vi "Event-Window.vi"(8 "error in (no error)":errorcluster, 9 "WindowEvent":T2, 10 "EventType":T1=enum."SDL_EVENT_WINDOW_DESTROYED", 11 "DVR Cluster In":T4={"CMD Queue"=refnum, "Config"={"Quit On Last Window Closed"=FALSE, "VSync"=enum."Disabled", "FPS Target"=30.0}, "Ctxt"={"VSync Enabled"=FALSE}, "Metrics"={"Uptime [ms]"=0, "Loop Time [ms]"=0, "Timer [ns]"=0, "Poll Events [ns]"=0, "Dequeue CMD [ns]"=0, "Update Layout [ns]"=0, "Render [ns]"=0}, "Debug"={"Unhandled Events"={}}, "ID To Window"={}, "Window To Handle"={}, "Event Interface"=refnum}) -> (0 "error out":errorcluster, 3 "DVR Cluster Out":T4={"CMD Queue"=refnum, "Config"={"Quit On Last Window Closed"=FALSE, "VSync"=enum."Disabled", "FPS Target"=30.0}, "Ctxt"={"VSync Enabled"=FALSE}, "Metrics"={"Uptime [ms]"=0, "Loop Time [ms]"=0, "Timer [ns]"=0, "Poll Events [ns]"=0, "Dequeue CMD [ns]"=0, "Update Layout [ns]"=0, "Render [ns]"=0}, "Debug"={"Unhandled Events"={}}, "ID To Window"={}, "Window To Handle"={}, "Event Interface"=refnum})   [LabVIEW 2020, in "GLF.lvlib" / "Engine.lvclass"]
uses:
  Engine.lvclass
  EngineEventInterface/EngineEventInterface.lvclass
  Window/Window.lvclass
  Engine.lvclass/Engine.ctl
  <vilib>/Utility/miscctls.llb/LVMapReplaceAction.ctl
  <vilib>/Saukko/LV SDL3/Sources/SDL3/Events/EventType--enum.ctl
  <vilib>/Saukko/LV SDL3/Sources/SDL3/Events/Events.lvlib
  <vilib>/Saukko/LV SDL3/Sources/SDL3/Video/DisplayID--integer.ctl
  <vilib>/Saukko/LV SDL3/Sources/SDL3/Video/Video.lvlib
  VSync--enum.ctl
  Config--cluster.ctl
  Context--cluster.ctl
  Metrics--cluster.ctl
  Command--enum.ctl
  Command--cluster.ctl
  Command--queue.ctl
  <vilib>/Saukko/LV SDL3/Sources/SDL3/Video/WindowID--integer.ctl
  DVR--cluster.ctl
  <vilib>/Saukko/LV SDL3/Sources/SDL3/Events/WindowEventData--cluster.ctl
  Debug--cluster.ctl
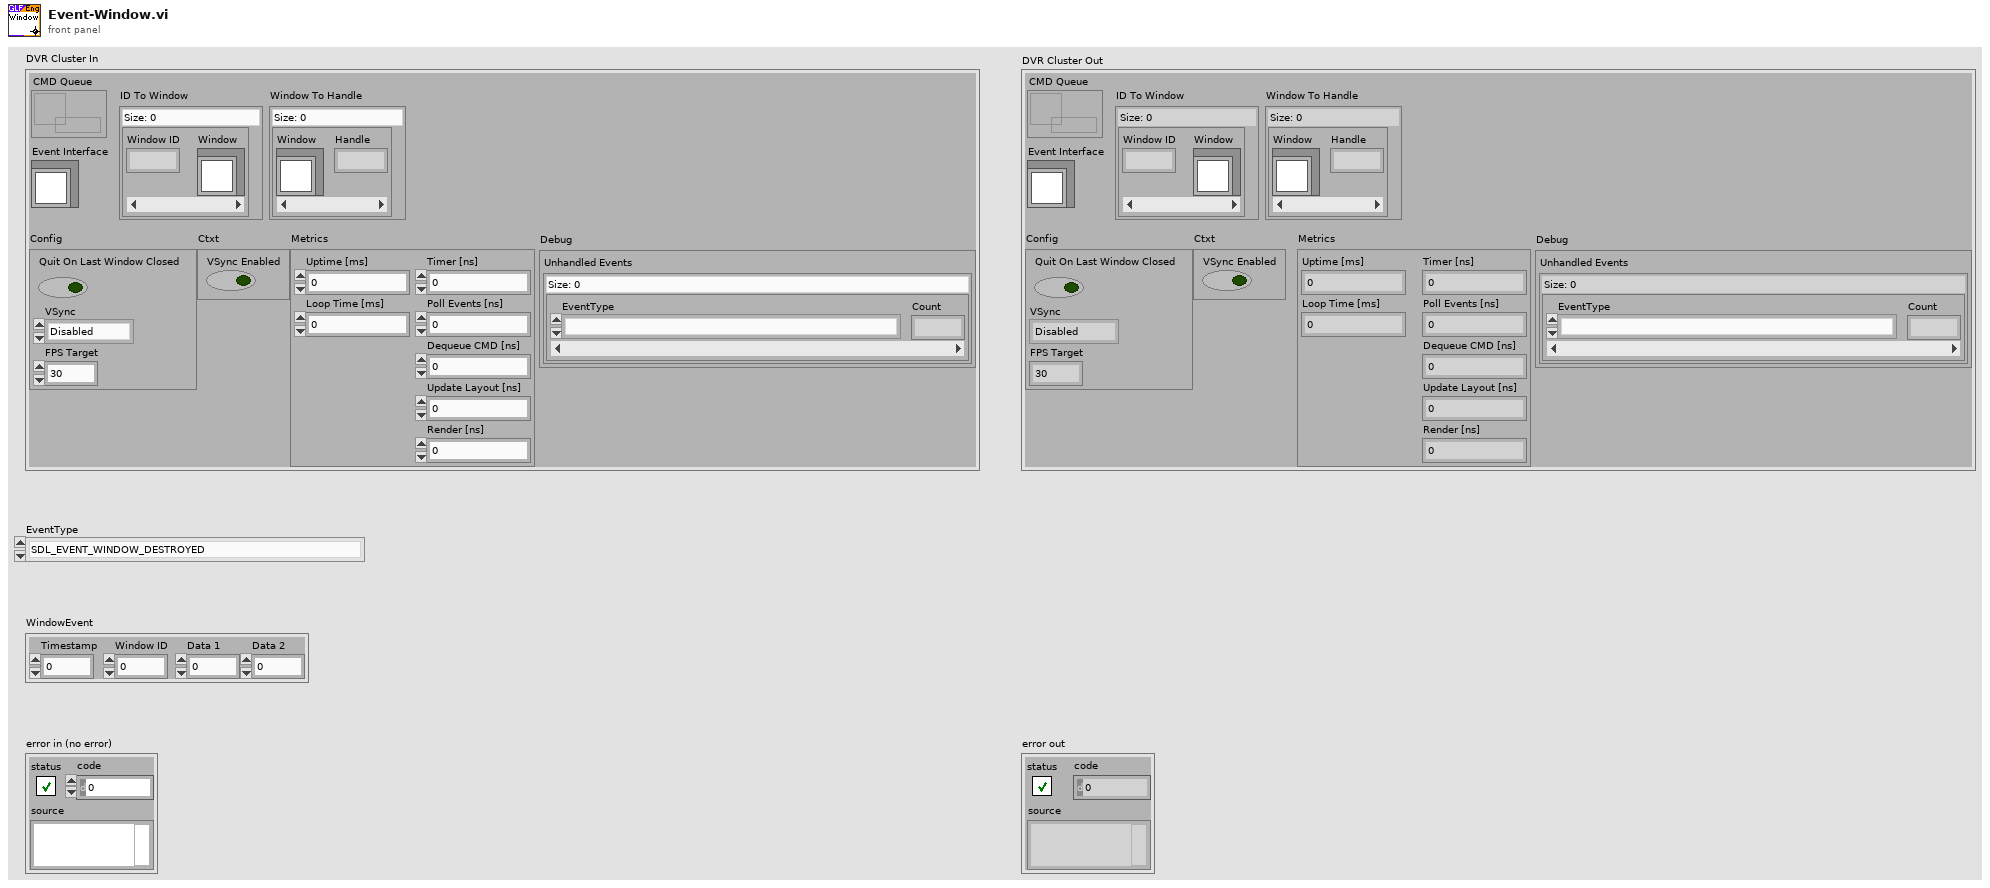
[diagram p1: front panel]
types:
  T1 = typedef "SDL3.lvlib/Events.lvlib/EventType--enum.ctl" = enum16{"LV_NONE", "LV_UNSUPPORTED", "SDL_EVENT_QUIT", "SDL_EVENT_LOCALE_CHANGED", "SDL_EVENT_SYSTEM_THEME_CHANGED", "SDL_EVENT_DISPLAY_ORIENTATION", "SDL_EVENT_DISPLAY_ADDED", "SDL_EVENT_DISPLAY_REMOVED", "SDL_EVENT_DISPLAY_MOVED", "SDL_EVENT_DISPLAY_DESKTOP_MODE_CHANGED", "SDL_EVENT_DISPLAY_CURRENT_MODE_CHANGED", "SDL_EVENT_DISPLAY_CONTENT_SCALE_CHANGED", "SDL_EVENT_WINDOW_SHOWN", "SDL_EVENT_WINDOW_HIDDEN", "SDL_EVENT_WINDOW_EXPOSED", "SDL_EVENT_WINDOW_MOVED", "SDL_EVENT_WINDOW_RESIZED", "SDL_EVENT_WINDOW_PIXEL_SIZE_CHANGED", "SDL_EVENT_WINDOW_METAL_VIEW_RESIZED", "SDL_EVENT_WINDOW_MINIMIZED", "SDL_EVENT_WINDOW_MAXIMIZED", "SDL_EVENT_WINDOW_RESTORED", "SDL_EVENT_WINDOW_MOUSE_ENTER", "SDL_EVENT_WINDOW_MOUSE_LEAVE", "SDL_EVENT_WINDOW_FOCUS_GAINED", "SDL_EVENT_WINDOW_FOCUS_LOST", "SDL_EVENT_WINDOW_CLOSE_REQUESTED", "SDL_EVENT_WINDOW_HIT_TEST", "SDL_EVENT_WINDOW_ICCPROF_CHANGED", "SDL_EVENT_WINDOW_DISPLAY_CHANGED", "SDL_EVENT_WINDOW_DISPLAY_SCALE_CHANGED", "SDL_EVENT_WINDOW_SAFE_AREA_CHANGED", "SDL_EVENT_WINDOW_OCCLUDED", "SDL_EVENT_WINDOW_ENTER_FULLSCREEN", "SDL_EVENT_WINDOW_LEAVE_FULLSCREEN", "SDL_EVENT_WINDOW_DESTROYED", "SDL_EVENT_WINDOW_HDR_STATE_CHANGED", "SDL_EVENT_KEY_DOWN", "SDL_EVENT_KEY_UP", "SDL_EVENT_TEXT_EDITING", "SDL_EVENT_TEXT_INPUT", "SDL_EVENT_KEYMAP_CHANGED", "SDL_EVENT_KEYBOARD_ADDED", "SDL_EVENT_KEYBOARD_REMOVED", "SDL_EVENT_TEXT_EDITING_CANDIDATES", "SDL_EVENT_MOUSE_MOTION", "SDL_EVENT_MOUSE_BUTTON_DOWN", "SDL_EVENT_MOUSE_BUTTON_UP", "SDL_EVENT_MOUSE_WHEEL", "SDL_EVENT_MOUSE_ADDED", "SDL_EVENT_MOUSE_REMOVED", "SDL_EVENT_JOYSTICK_AXIS_MOTION", "SDL_EVENT_JOYSTICK_BALL_MOTION", "SDL_EVENT_JOYSTICK_HAT_MOTION", "SDL_EVENT_JOYSTICK_BUTTON_DOWN", "SDL_EVENT_JOYSTICK_BUTTON_UP", "SDL_EVENT_JOYSTICK_ADDED", "SDL_EVENT_JOYSTICK_REMOVED", "SDL_EVENT_JOYSTICK_BATTERY_UPDATED", "SDL_EVENT_JOYSTICK_UPDATE_COMPLETE", "SDL_EVENT_GAMEPAD_AXIS_MOTION", "SDL_EVENT_GAMEPAD_BUTTON_DOWN", "SDL_EVENT_GAMEPAD_BUTTON_UP", "SDL_EVENT_GAMEPAD_ADDED", "SDL_EVENT_GAMEPAD_REMOVED", "SDL_EVENT_GAMEPAD_REMAPPED", "SDL_EVENT_GAMEPAD_TOUCHPAD_DOWN", "SDL_EVENT_GAMEPAD_TOUCHPAD_MOTION", "SDL_EVENT_GAMEPAD_TOUCHPAD_UP", "SDL_EVENT_GAMEPAD_SENSOR_UPDATE", "SDL_EVENT_GAMEPAD_UPDATE_COMPLETE", "SDL_EVENT_GAMEPAD_STEAM_HANDLE_UPDATED", "SDL_EVENT_FINGER_DOWN", "SDL_EVENT_FINGER_UP", "SDL_EVENT_FINGER_MOTION", "SDL_EVENT_CLIPBOARD_UPDATE", "SDL_EVENT_DROP_FILE", "SDL_EVENT_DROP_TEXT", "SDL_EVENT_DROP_BEGIN", "SDL_EVENT_DROP_COMPLETE", "SDL_EVENT_DROP_POSITION", "SDL_EVENT_AUDIO_DEVICE_ADDED", "SDL_EVENT_AUDIO_DEVICE_REMOVED", "SDL_EVENT_AUDIO_DEVICE_FORMAT_CHANGED", "SDL_EVENT_SENSOR_UPDATE", "SDL_EVENT_PEN_PROXIMITY_IN", "SDL_EVENT_PEN_PROXIMITY_OUT", "SDL_EVENT_PEN_DOWN", "SDL_EVENT_PEN_UP", "SDL_EVENT_PEN_BUTTON_DOWN", "SDL_EVENT_PEN_BUTTON_UP", "SDL_EVENT_PEN_MOTION", "SDL_EVENT_PEN_AXIS", "SDL_EVENT_CAMERA_DEVICE_ADDED", "SDL_EVENT_CAMERA_DEVICE_REMOVED", "SDL_EVENT_CAMERA_DEVICE_APPROVED", "SDL_EVENT_CAMERA_DEVICE_DENIED", "SDL_EVENT_RENDER_TARGETS_RESET", "SDL_EVENT_RENDER_DEVICE_RESET", "SDL_EVENT_POLL_SENTINEL", "SDL_EVENT_USER"}
  T2 = typedef "SDL3.lvlib/Events.lvlib/WindowEventData--cluster.ctl" = cluster{"Timestamp":u64, "Window ID":T3, "Data 1":i32, "Data 2":i32}
  T3 = typedef "SDL3.lvlib/Video.lvlib/WindowID--integer.ctl" = u32
  T4 = typedef "GLF.lvlib/Engine.lvclass/DVR--cluster.ctl" = cluster{"CMD Queue":T5, "Config":T6, "Ctxt":T8, "Metrics":T9, "Debug":T10, "ID To Window":map{T3, refnum<class "Window.lvclass">}, "Window To Handle":map{refnum<class "Window.lvclass">, i64}, "Event Interface":refnum<class "EngineEventInterface.lvclass">}
  T5 = typedef "GLF.lvlib/Engine.lvclass/Command--queue.ctl" = refnum<queue>
  T6 = typedef "GLF.lvlib/Engine.lvclass/Config--cluster.ctl" = cluster{"Quit On Last Window Closed":bool, "VSync":T7, "FPS Target":dbl}
  T7 = typedef "GLF.lvlib/Engine.lvclass/VSync--enum.ctl" = enum16{"Disabled", "Enabled", "Adaptative"}
  T8 = typedef "GLF.lvlib/Engine.lvclass/Context--cluster.ctl" = cluster{"VSync Enabled":bool}
  T9 = typedef "GLF.lvlib/Engine.lvclass/Metrics--cluster.ctl" = cluster{"Uptime [ms]":u64, "Loop Time [ms]":u64, "Timer [ns]":u64, "Poll Events [ns]":u64, "Dequeue CMD [ns]":u64, "Update Layout [ns]":u64, "Render [ns]":u64}
  T10 = typedef "GLF.lvlib/Engine.lvclass/Debug--cluster.ctl" = cluster{"Unhandled Events":map{T1, u64}}
  T11 = typedef "LVMapReplaceAction.ctl" = enum32{"Modify Entry only if found", "Add or Modify Entry", "Delete Entry"}
  T12 = typedef "SDL3.lvlib/Video.lvlib/DisplayID--integer.ctl" = u32
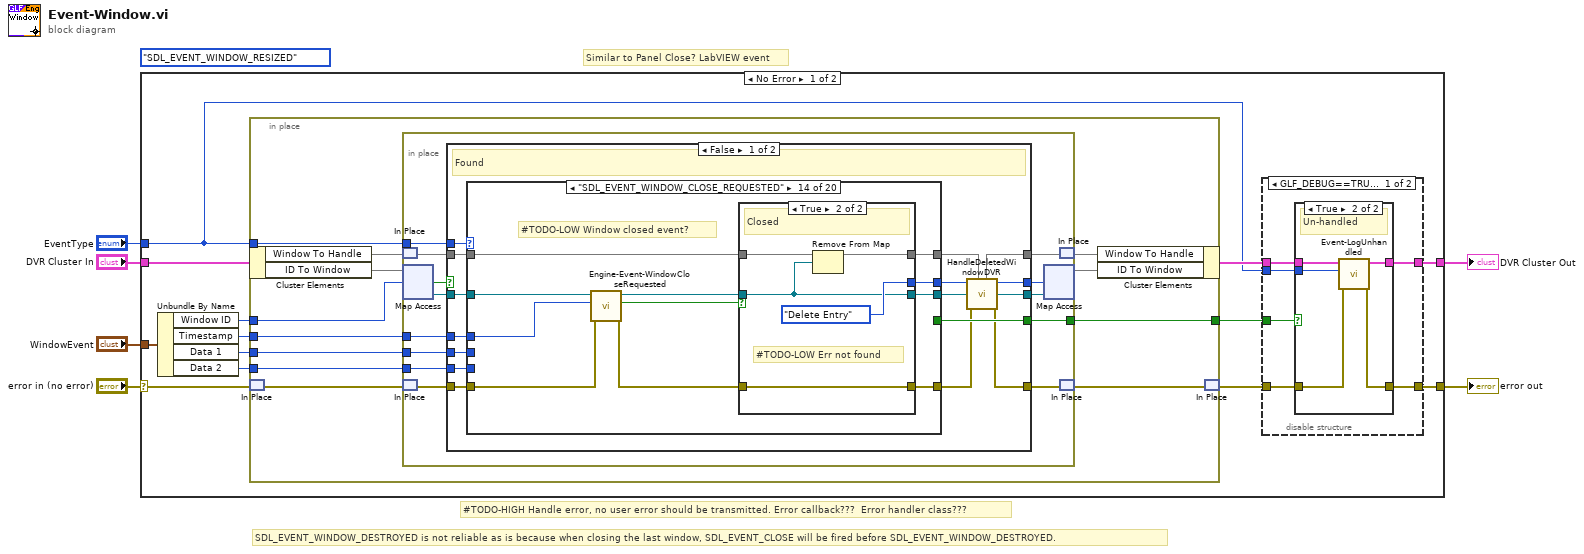
[diagram p0: block diagram]
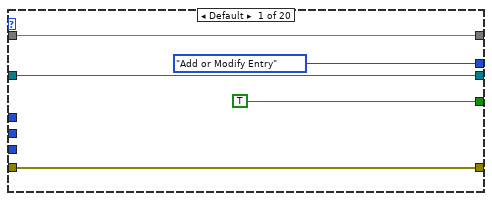
[diagram p2: hidden frame]
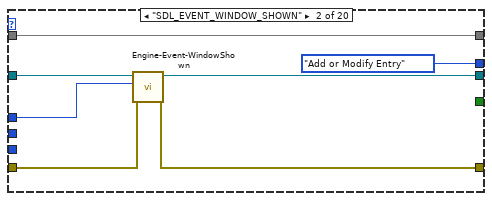
[diagram p3: hidden frame]
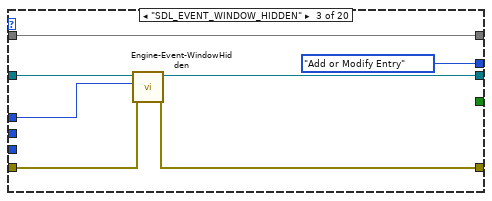
[diagram p4: hidden frame]
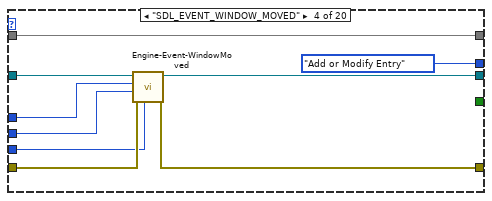
[diagram p5: hidden frame]
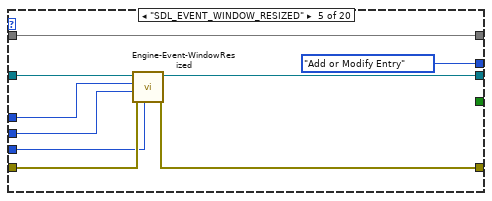
[diagram p6: hidden frame]
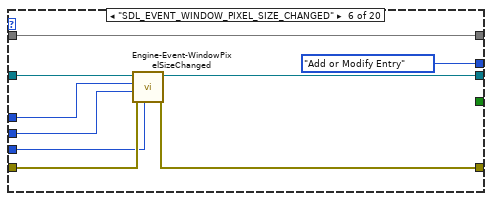
[diagram p7: hidden frame]
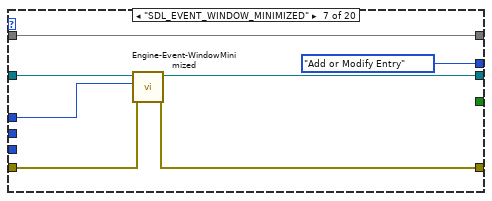
[diagram p8: hidden frame]
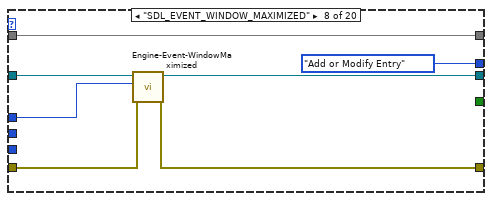
[diagram p9: hidden frame]
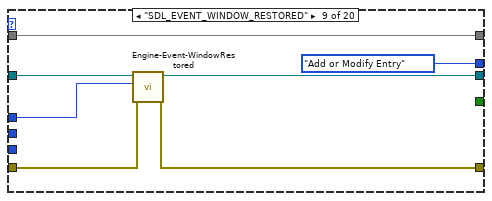
[diagram p10: hidden frame]
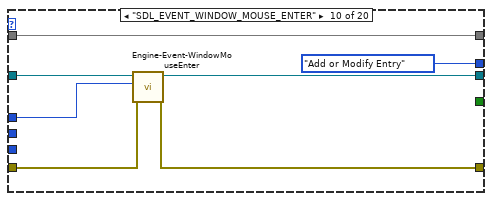
[diagram p11: hidden frame]
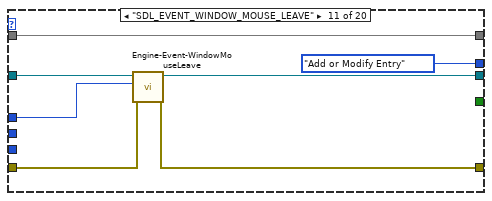
[diagram p12: hidden frame]
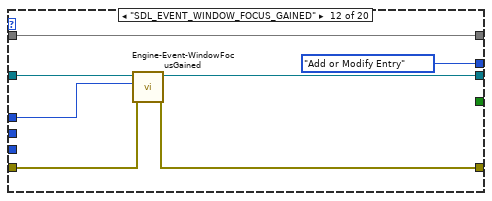
[diagram p13: hidden frame]
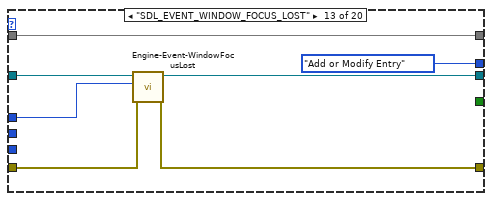
[diagram p14: hidden frame]
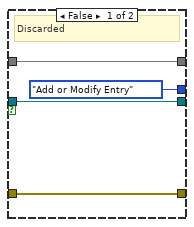
[diagram p15: hidden frame]
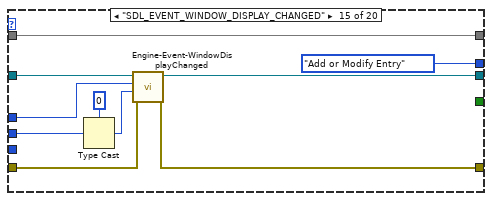
[diagram p16: hidden frame]
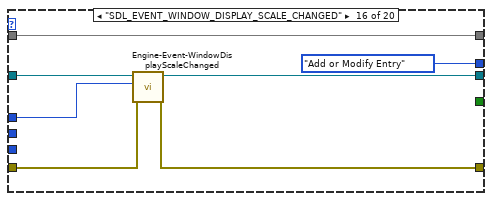
[diagram p17: hidden frame]
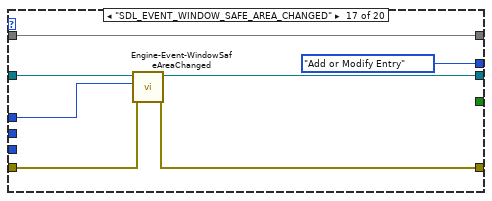
[diagram p18: hidden frame]
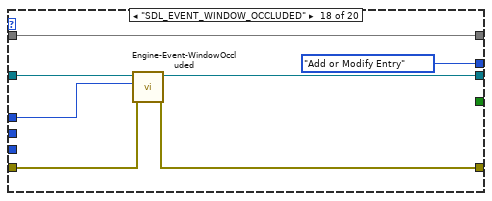
[diagram p19: hidden frame]
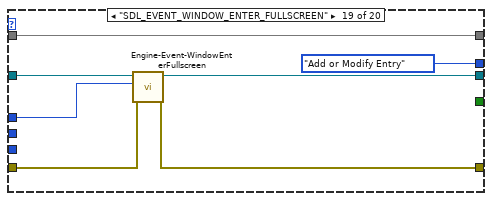
[diagram p20: hidden frame]
diagram:
  (unwired) EventType--enum."SDL_EVENT_WINDOW_RESIZED" ("EventType")
  # "SDL_EVENT_WINDOW_DESTROYED is not reliable as is because when closing the last window, SDL_EVENT_CLOSE will be fired before SDL_EVENT_WINDOW_DESTROYED."
  # "#TODO-HIGH Handle error, no user error should be transmitted. Error callback???  Error handler class???"
  # "Similar to Panel Close? LabVIEW event"
  n1 = case shown="No Error" "error in (no error)" {
    selector: "error in (no error)" -> [w16 w240]
    tunnel: [w11 w240] -> w5
    tunnel: [w12 w239] -> w3
    tunnel: "DVR Cluster In" -> [w18 w239]
    tunnel: "WindowEvent" -> [w19 _]
    tunnel: "EventType" -> [w10 _]
    frame No Error {
      n2 = Unbundle By Name(w19) -> ("Window ID"=w17:T3, "Timestamp"=w15:u64, "Data 1"=w8:i32, "Data 2"=w7:i32)
      n3 = in-place {
        in-place-border: w17 -> [w30]
        in-place-border: w15 -> [w27]
        in-place-border: w10 -> [w25]
        in-place-border: [w24] -> w9
        in-place-border: w8 -> [w23]
        in-place-border: w7 -> [w22]
        n4 = in-place-cluster #1(w18) -> ("Window To Handle"=w21:map{refnum<class "Window.lvclass">, i64}, "ID To Window"=w31:map{T3, refnum<class "Window.lvclass">})
        n5 = in-place-match #2(w16) -> (w29:errorcluster)
        n6 = in-place {
          in-place-border: w27 -> [w38]
          in-place-border: w25 -> [w37]
          in-place-border: [w36] -> w24
          in-place-border: w23 -> [w35]
          in-place-border: w22 -> [w34]
          n7 = in-place-match #3(w21) -> (w33:map{refnum<class "Window.lvclass">, i64})
          n8 = in-place-map #4(w31, w30) -> (w43:refnum<class "Window.lvclass">, w44:bool)  [unwired: 1 in]
          n9 = in-place-match #5(w29) -> (w41:errorcluster)
          n10 = case shown="False" w44 {
            tunnel: w43 -> [w59 w221]
            tunnel: [w46 LVMapReplaceAction."Modify Entry only if found" ("Replace Action")] -> w42
            tunnel: [w53 w222] -> w40
            tunnel: w41 -> [w58 w222]
            tunnel: [w45 w221] -> w39
            tunnel: w38 -> [w57 _]
            tunnel: w37 -> [w56 _]
            tunnel: [w55 _] -> w36
            tunnel: w35 -> [w52 _]
            tunnel: w34 -> [w51 _]
            tunnel: w33 -> [w50 w220]
            tunnel: [w49 w220] -> w32
            frame False {
              # "Found"
              n11 = case shown="\"SDL_EVENT_WINDOW_CLOSE_REQUESTED\"" w56 {
                tunnel: [w61 w71 w78 w87 w96 w105 w112 w119 w126 w133 w140 w147 w154 w165 w184 w191 w198 w205 w212 w219] -> w54
                tunnel: [w62 w70 w77 w86 w95 w104 w111 w118 w125 w132 w139 w146 w153 w164 w183 w190 w197 w204 w211 w218] -> w45
                tunnel: [LVMapReplaceAction."Add or Modify Entry" ("Replace Action") LVMapReplaceAction."Add or Modify Entry" ("Replace Action") LVMapReplaceAction."Add or Modify Entry" ("Replace Action") LVMapReplaceAction."Add or Modify Entry" ("Replace Action") LVMapReplaceAction."Add or Modify Entry" ("Replace Action") LVMapReplaceAction."Add or Modify Entry" ("Replace Action") LVMapReplaceAction."Add or Modify Entry" ("Replace Action") LVMapReplaceAction."Add or Modify Entry" ("Replace Action") LVMapReplaceAction."Add or Modify Entry" ("Replace Action") LVMapReplaceAction."Add or Modify Entry" ("Replace Action") LVMapReplaceAction."Add or Modify Entry" ("Replace Action") LVMapReplaceAction."Add or Modify Entry" ("Replace Action") LVMapReplaceAction."Add or Modify Entry" ("Replace Action") w163 LVMapReplaceAction."Add or Modify Entry" ("Replace Action") LVMapReplaceAction."Add or Modify Entry" ("Replace Action") LVMapReplaceAction."Add or Modify Entry" ("Replace Action") LVMapReplaceAction."Add or Modify Entry" ("Replace Action") LVMapReplaceAction."Add or Modify Entry" ("Replace Action") LVMapReplaceAction."Add or Modify Entry" ("Replace Action")] -> w47
                tunnel: w59 -> [w62 w67 w74 w83 w92 w101 w108 w115 w122 w129 w136 w143 w150 w160 w180 w187 w194 w201 w208 w215]
                tunnel: w58 -> [w61 w66 w73 w82 w91 w100 w107 w114 w121 w128 w135 w142 w149 w159 w179 w186 w193 w200 w207 w214]
                tunnel: w57 -> [_ w65 w72 w81 w90 w99 w106 w113 w120 w127 w134 w141 w148 w155 w178 w185 w192 w199 w206 w213]
                tunnel: [TRUE _ _ _ _ _ _ _ _ _ _ _ _ _ _ _ _ _ _ _] -> w55
                tunnel: w52 -> [_ _ _ w80 w89 w98 _ _ _ _ _ _ _ _ w177 _ _ _ _ _]
                tunnel: w51 -> [_ _ _ w79 w88 w97 _ _ _ _ _ _ _ _ _ _ _ _ _ _]
                tunnel: w50 -> [w60 w68 w75 w84 w93 w102 w109 w116 w123 w130 w137 w144 w151 w161 w181 w188 w195 w202 w209 w216]
                tunnel: [w60 w68 w75 w84 w93 w102 w109 w116 w123 w130 w137 w144 w151 w162 w181 w188 w195 w202 w209 w216] -> w48
                frame Default {
                }
                frame "SDL_EVENT_WINDOW_SHOWN" {
                  n12 = call "Engine-Event-WindowShown.vi"("error in (no error)"=w66, "Timestamp"=w65, "GLF Window in"=w67) -> ("error out"=w71:errorcluster, "GLF Window out"=w70:refnum<class "Window.lvclass">)  [unwired: 7 in]
                }
                frame "SDL_EVENT_WINDOW_HIDDEN" {
                  n13 = call "Engine-Event-WindowHidden.vi"("error in (no error)"=w73, "Timestamp"=w72, "GLF Window in"=w74) -> ("error out"=w78:errorcluster, "GLF Window out"=w77:refnum<class "Window.lvclass">)  [unwired: 7 in]
                }
                frame "SDL_EVENT_WINDOW_MOVED" {
                  n14 = call "Engine-Event-WindowMoved.vi"("Y"=w79, "error in (no error)"=w82, "X"=w80, "Timestamp"=w81, "GLF Window in"=w83) -> ("error out"=w87:errorcluster, "GLF Window out"=w86:refnum<class "Window.lvclass">)  [unwired: 5 in]
                }
                frame "SDL_EVENT_WINDOW_RESIZED" {
                  n15 = call "Engine-Event-WindowResized.vi"("Height"=w88, "error in (no error)"=w91, "Width"=w89, "Timestamp"=w90, "GLF Window in"=w92) -> ("error out"=w96:errorcluster, "GLF Window out"=w95:refnum<class "Window.lvclass">)  [unwired: 5 in]
                }
                frame "SDL_EVENT_WINDOW_PIXEL_SIZE_CHANGED" {
                  n16 = call "Engine-Event-WindowPixelSizeChanged.vi"("Height"=w97, "error in (no error)"=w100, "Width"=w98, "Timestamp"=w99, "GLF Window in"=w101) -> ("error out"=w105:errorcluster, "GLF Window out"=w104:refnum<class "Window.lvclass">)  [unwired: 5 in]
                }
                frame "SDL_EVENT_WINDOW_MINIMIZED" {
                  n17 = call "Engine-Event-WindowMinimized.vi"("error in (no error)"=w107, "Timestamp"=w106, "GLF Window in"=w108) -> ("error out"=w112:errorcluster, "GLF Window out"=w111:refnum<class "Window.lvclass">)  [unwired: 7 in]
                }
                frame "SDL_EVENT_WINDOW_MAXIMIZED" {
                  n18 = call "Engine-Event-WindowMaximized.vi"("error in (no error)"=w114, "Timestamp"=w113, "GLF Window in"=w115) -> ("error out"=w119:errorcluster, "GLF Window out"=w118:refnum<class "Window.lvclass">)  [unwired: 7 in]
                }
                frame "SDL_EVENT_WINDOW_RESTORED" {
                  n19 = call "Engine-Event-WindowRestored.vi"("error in (no error)"=w121, "Timestamp"=w120, "GLF Window in"=w122) -> ("error out"=w126:errorcluster, "GLF Window out"=w125:refnum<class "Window.lvclass">)  [unwired: 7 in]
                }
                frame "SDL_EVENT_WINDOW_MOUSE_ENTER" {
                  n20 = call "Engine-Event-WindowMouseEnter.vi"("error in (no error)"=w128, "Timestamp"=w127, "GLF Window in"=w129) -> ("error out"=w133:errorcluster, "GLF Window out"=w132:refnum<class "Window.lvclass">)  [unwired: 7 in]
                }
                frame "SDL_EVENT_WINDOW_MOUSE_LEAVE" {
                  n21 = call "Engine-Event-WindowMouseLeave.vi"("error in (no error)"=w135, "Timestamp"=w134, "GLF Window in"=w136) -> ("error out"=w140:errorcluster, "GLF Window out"=w139:refnum<class "Window.lvclass">)  [unwired: 7 in]
                }
                frame "SDL_EVENT_WINDOW_FOCUS_GAINED" {
                  n22 = call "Engine-Event-WindowFocusGained.vi"("error in (no error)"=w142, "Timestamp"=w141, "GLF Window in"=w143) -> ("error out"=w147:errorcluster, "GLF Window out"=w146:refnum<class "Window.lvclass">)  [unwired: 7 in]
                }
                frame "SDL_EVENT_WINDOW_FOCUS_LOST" {
                  n23 = call "Engine-Event-WindowFocusLost.vi"("error in (no error)"=w149, "Timestamp"=w148, "GLF Window in"=w150) -> ("error out"=w154:errorcluster, "GLF Window out"=w153:refnum<class "Window.lvclass">)  [unwired: 7 in]
                }
                frame "SDL_EVENT_WINDOW_CLOSE_REQUESTED" {
                  # "#TODO-LOW Window closed event?"
                  n24 = call "Engine-Event-WindowCloseRequested.vi"("error in (no error)"=w159, "Timestamp"=w155, "GLF Window in"=w160) -> ("error out"=w158:errorcluster, "Closed?"=w157:bool, "GLF Window out"=w156:refnum<class "Window.lvclass">)  [unwired: 6 in]
                  n25 = case shown="True" w157 {
                    tunnel: w156 -> [w168 w170]
                    tunnel: w158 -> [w167 w173]
                    tunnel: [w167 w173] -> w165
                    tunnel: [w168 w170] -> w164
                    tunnel: [LVMapReplaceAction."Add or Modify Entry" ("Replace Action") LVMapReplaceAction."Delete Entry" ("Replace Action")] -> w163
                    tunnel: [w166 w171] -> w162
                    tunnel: w161 -> [w166 w172]
                    frame False {
                      # "Discarded"
                    }
                    frame True {
                      # "#TODO-LOW Err not found"
                      # "Closed"
                      n26 = Remove From Map(10:w170, 11:w172) -> (3:w171:map{refnum<class "Window.lvclass">, i64})  [unwired: 2 out]
                    }
                  }
                }
                frame "SDL_EVENT_WINDOW_DISPLAY_CHANGED" {
                  n27 = Type Cast(type=T12 0 ("Display ID"), x=w177) -> (*(type *) &x=w175:T12)
                  n28 = call "Engine-Event-WindowDisplayChanged.vi"("error in (no error)"=w179, "Display ID"=w175, "Timestamp"=w178, "GLF Window in"=w180) -> ("error out"=w184:errorcluster, "GLF Window out"=w183:refnum<class "Window.lvclass">)  [unwired: 6 in]
                }
                frame "SDL_EVENT_WINDOW_DISPLAY_SCALE_CHANGED" {
                  n29 = call "Engine-Event-WindowDisplayScaleChanged.vi"("error in (no error)"=w186, "Timestamp"=w185, "GLF Window in"=w187) -> ("error out"=w191:errorcluster, "GLF Window out"=w190:refnum<class "Window.lvclass">)  [unwired: 7 in]
                }
                frame "SDL_EVENT_WINDOW_SAFE_AREA_CHANGED" {
                  n30 = call "Engine-Event-WindowSafeAreaChanged.vi"("error in (no error)"=w193, "Timestamp"=w192, "GLF Window in"=w194) -> ("error out"=w198:errorcluster, "GLF Window out"=w197:refnum<class "Window.lvclass">)  [unwired: 7 in]
                }
                frame "SDL_EVENT_WINDOW_OCCLUDED" {
                  n31 = call "Engine-Event-WindowOccluded.vi"("error in (no error)"=w200, "Timestamp"=w199, "GLF Window in"=w201) -> ("error out"=w205:errorcluster, "GLF Window out"=w204:refnum<class "Window.lvclass">)  [unwired: 7 in]
                }
                frame "SDL_EVENT_WINDOW_ENTER_FULLSCREEN" {
                  n32 = call "Engine-Event-WindowEnterFullscreen.vi"("error in (no error)"=w207, "Timestamp"=w206, "GLF Window in"=w208) -> ("error out"=w212:errorcluster, "GLF Window out"=w211:refnum<class "Window.lvclass">)  [unwired: 7 in]
                }
                frame "SDL_EVENT_WINDOW_LEAVE_FULLSCREEN" {
                  n33 = call "Engine-Event-WindowLeaveFullscreen.vi"("error in (no error)"=w214, "Timestamp"=w213, "GLF Window in"=w215) -> ("error out"=w219:errorcluster, "GLF Window out"=w218:refnum<class "Window.lvclass">)  [unwired: 7 in]
                }
              }
              n34 = call "HandleDeletedWindowDVR.vi"("Window To Handle In"=w48, "error in (no error)"=w54, "Window"=w45, "Replace Action In"=w47) -> ("error out"=w53:errorcluster, "Replace Action Out"=w46:T11, "Window To Handle Out"=w49:map{refnum<class "Window.lvclass">, i64})  [unwired: 5 in]
            }
            frame True {
              # "#TODO-MEDIUM Window not found\nMaybe the window has been closed since the last event loop?"
              # "Not found"
            }
          }
          n35 = in-place-map #4(w39, w42) -> (w26:map{T3, refnum<class "Window.lvclass">})  [unwired: 2 out]
          n36 = in-place-match #3(w32) -> (w20:map{refnum<class "Window.lvclass">, i64})
          n37 = in-place-match #5(w40) -> (w28:errorcluster)
        }
        n38 = in-place-cluster #1("Window To Handle"=w20, "ID To Window"=w26) -> (w13:T4)
        n39 = in-place-match #2(w28) -> (w14:errorcluster)
      }
      n40 = disable-structure shown="GLF_DEBUG==TRUE" {
        disable-tunnel: w14 -> [w229 w237]
        disable-tunnel: w13 -> [w228 w238]
        disable-tunnel: [w227 w238] -> w12
        disable-tunnel: [w226 w237] -> w11
        disable-tunnel: w10 -> [w225 _]
        disable-tunnel: w9 -> [w224 _]
        frame condition #0 (active) {
          n41 = case shown="True" w224 {
            tunnel: w229 -> [w230 w236]
            tunnel: w228 -> [w231 w235]
            tunnel: [w231 w234] -> w227
            tunnel: [w230 w233] -> w226
            tunnel: w225 -> [_ w232]
            frame False {
              # "Handled"
            }
            frame True {
              # "Un-handled"
              n42 = call "Event-LogUnhandled.vi"("error in (no error)"=w236, "EventType"=w232, "DVR Cluster In"=w235) -> ("error out"=w233:errorcluster, "DVR Cluster Out"=w234:T4)  [unwired: 7 in]
            }
          }
        }
        frame condition #1 {
        }
      }
    }
    frame Error {
    }
  }
  "error out" <- w5
  "DVR Cluster Out" <- w3
